vi "Read Repeat times.vi"(8 "error in (no error)":errorcluster, 11 "Process Controller in":refnum<class "Process Controller.lvclass">) -> (0 "error out":errorcluster, 2 "Repeat times":i32, 3 "Process Controller out":refnum<class "Process Controller.lvclass">)   [LabVIEW 2016, in "Process Controller.lvclass"]
uses:
  Process Controller.lvclass
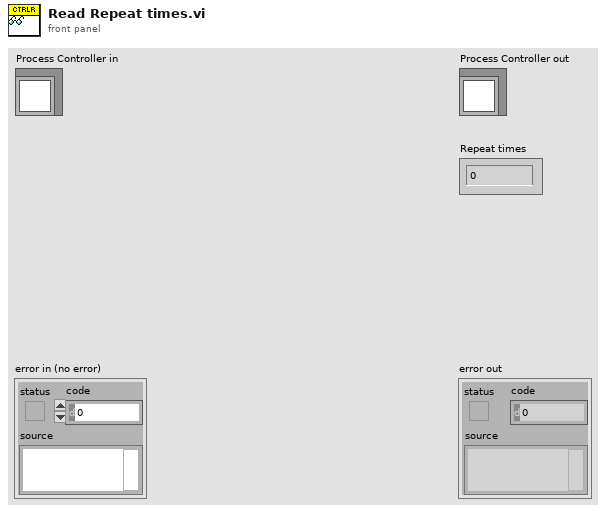
[diagram p1: front panel]
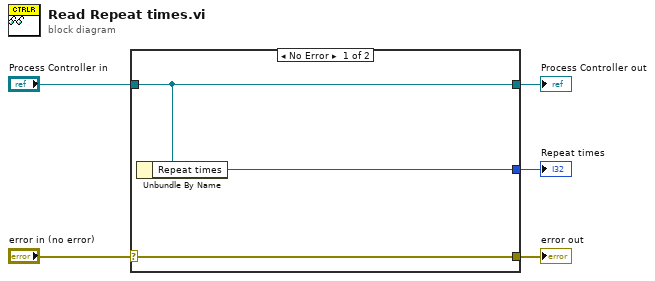
[diagram p0: block diagram]
diagram:
  n1 = case shown="No Error" "error in (no error)" {
    selector: "error in (no error)" -> [w8 w9]
    tunnel: [w8 w9] -> w4
    tunnel: [w7 w10] -> w2
    tunnel: "Process Controller in" -> [w7 w10]
    tunnel: [w6 _] -> w1
    frame No Error {
      n2 = Unbundle By Name(w7) -> ("Repeat times"=w6:i32)
    }
    frame Error {
    }
  }
  "error out" <- w4
  "Process Controller out" <- w2
  "Repeat times" <- w1
